vi "from string.vi"(8 "error in":errorcluster, 9 "data":string, 10 "version":string, 11 "Shared Library Module configuration in":refnum<class "Shared Library Module configuration.lvclass">) -> (0 "error out":errorcluster, 3 "Shared Library Module configuration out":refnum<class "Shared Library Module configuration.lvclass">)   [LabVIEW 2013, in "Shared Library Module configuration.lvclass"]
doc: "Provides an interface for loading a module configuration from a file or other serialized data source. It is recommended that all children of this class store data in two sets--data required for its own initialization, and any data required for parent initialization--and that each implementation uses the <b>Call Parent Method</b> primitive to de-serialize parent information. As a result, it is expected that every module configuration class calls <b>component configuration.lvclass:From String.vi</b>.Platypus Framework 1.0.1.60\nNI Systems Engineering - National Instruments"
uses:
  Shared Library Module configuration.lvclass
  <vilib>/NI/Tag Bus Module Framework/channel/TBM channel.lvclass
  <vilib>/NI/Tag Bus Module Framework/module configuration/TBM module configuration.lvclass
  Shared Library Module configuration.lvclass/Shared Library Module configuration.ctl
  <vilib>/NI/Configuration Framework/serializable configuration/NISE_CEF_serializable configuration.lvclass
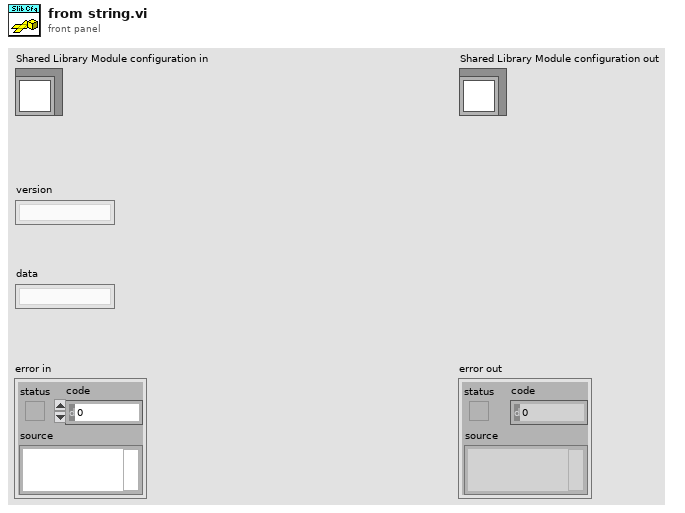
[diagram p1: front panel]
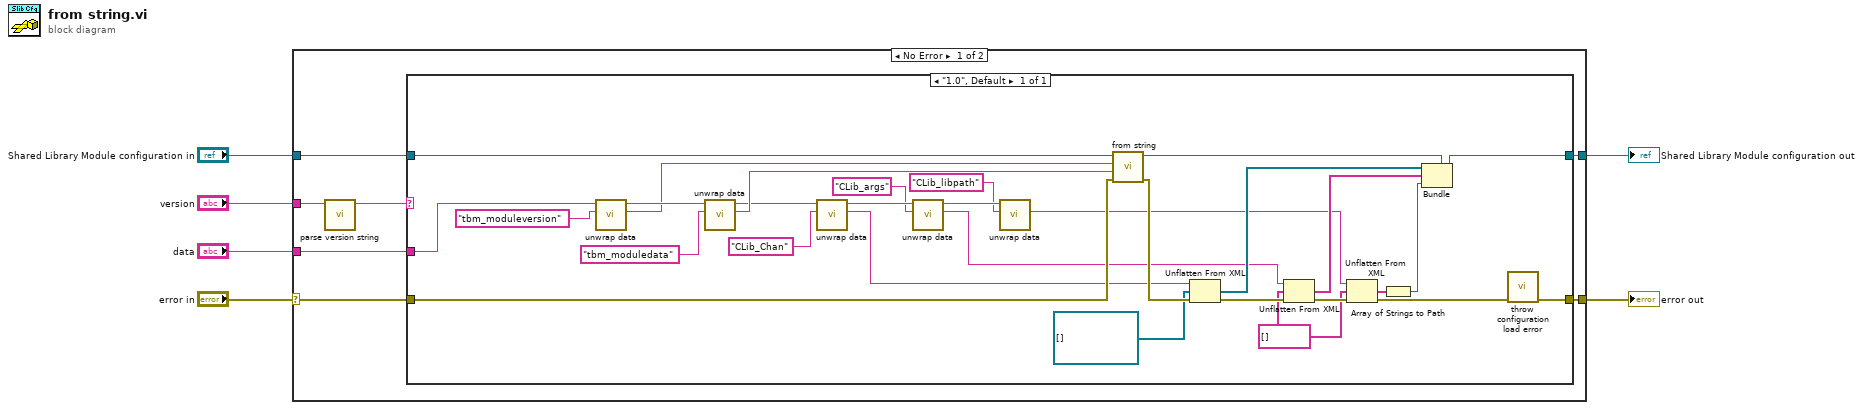
[diagram p0: block diagram]
diagram:
  n1 = case shown="No Error" "error in" {
    selector: "error in" -> [w7 w45]
    tunnel: "data" -> [w13 _]
    tunnel: "Shared Library Module configuration in" -> [w12 w44]
    tunnel: [w11 w44] -> w2
    tunnel: [w10 w45] -> w1
    tunnel: "version" -> [w9 _]
    frame No Error {
      n2 = call <vilib>:"parse version string.vi"("full version"=w9) -> ("major.minor version"=w8:string)  [unwired: 7 in, 3 out]
      n3 = case shown="\"1.0\", Default" w8 {
        tunnel: w13 -> [w38]
        tunnel: w7 -> [w37]
        tunnel: w12 -> [w43]
        tunnel: [w32] -> w11
        tunnel: [w40] -> w10
        frame "1.0", Default {
          w24 = string[] [] ("array of strings")
          n4 = call <vilib>:"unwrap data.vi"("identifier"="tbm_moduleversion" ("additional identifier"), "data to unwrap"=w38) -> ("unwrapped data"=w33:string, "remaining string"=w39:string)  [unwired: 8 in]
          n5 = call <vilib>:"unwrap data.vi"("identifier"="tbm_moduledata" ("additional identifier"), "data to unwrap"=w39) -> ("unwrapped data"=w35:string, "remaining string"=w28:string)  [unwired: 8 in]
          n6 = call <vilib>:"unwrap data.vi"("identifier"="CLib_Chan" ("additional identifier"), "data to unwrap"=w28) -> ("unwrapped data"=w27:string, "remaining string"=w20:string)  [unwired: 8 in]
          n7 = call <vilib>:"unwrap data.vi"("identifier"="CLib_args" ("additional identifier"), "data to unwrap"=w20) -> ("unwrapped data"=w15:string, "remaining string"=w19:string)  [unwired: 8 in]
          n8 = call <vilib>:"unwrap data.vi"("identifier"="CLib_libpath" ("additional identifier"), "data to unwrap"=w19) -> ("unwrapped data"=w14:string)  [unwired: 8 in, 1 out]
          n9 = call-parent "from string.vi"("error in"=w37, "data"=w35, "version"=w33, "module configuration in"=w43) -> ("error out"=w41:errorcluster, "module configuration out"=w42:refnum<class "Shared Library Module configuration.lvclass">)  [unwired: 6 in]
          n10 = Unflatten From XML(xml string=w27, type=refnum<class "TBM channel.lvclass">[] [] ("channels"), error in (no error)=w41) -> (value=w29:refnum<class "TBM channel.lvclass">[], error out=w31:errorcluster)
          n11 = Unflatten From XML(xml string=w15, type=w24, error in (no error)=w31) -> (value=w21:string[], error out=w25:errorcluster)
          n12 = Unflatten From XML(xml string=w14, type=w24, error in (no error)=w25) -> (value=w23:string[], error out=w26:errorcluster)
          n13 = Array of Strings to Path(0:w23) -> (2:w22:path)  [unwired: 1 in]
          n14 = Bundle(cluster=w42, w29, w21, w22) -> (w32:refnum<class "Shared Library Module configuration.lvclass">)
          n15 = call <vilib>:"throw configuration load error.vi"("error in"=w26) -> ("error out"=w40:errorcluster)  [unwired: 10 in]
        }
      }
    }
    frame Error {
    }
  }
  "error out" <- w1
  "Shared Library Module configuration out" <- w2
